vi "getAllAttributes.vi"(8 "error in (no error)":errorcluster, 11 "NativeXML in":refnum<class "NativeXML.lvclass">) -> (0 "error out":errorcluster, 1 "values":string[](array[string]), 2 "names":string[](array[string]), 3 "NativeXML out":refnum<class "NativeXML.lvclass">)   [LabVIEW 2009, in "Tools.lvlib" / "xml.lvlib" / "NativeXML.lvclass"]
uses:
  NativeXML.lvclass
  NativeXML.lvclass/NativeXML.ctl
  <vilib>/xml/Close Reference(NNMap).vi
  <vilib>/xml/Close Reference(Node).vi
  Program Files/National Instruments/LabVIEW 2009/resource/objmgr/DOMUserDefRef.rc
  <vilib>/xml/NI_XML.lvlib
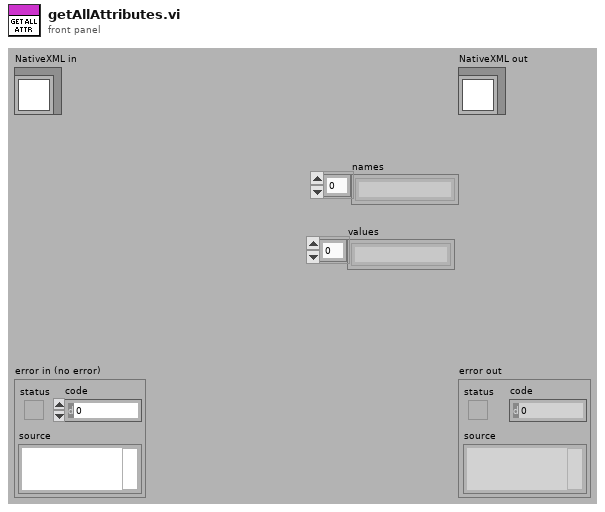
[diagram p1: front panel]
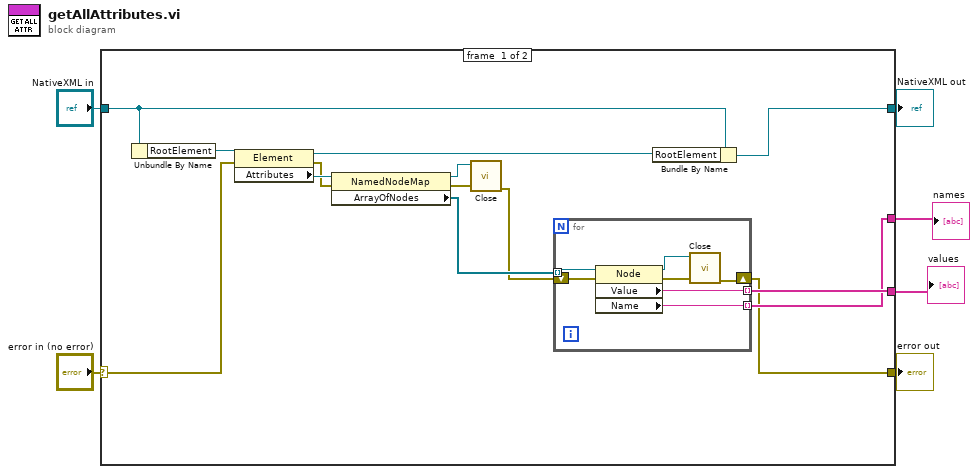
[diagram p0: block diagram]
diagram:
  n1 = case shown="No Error" "error in (no error)" {
    selector: "error in (no error)" -> [w12 w29]
    tunnel: [w14 w29] -> w5
    tunnel: [w19 w28] -> w3
    tunnel: "NativeXML in" -> [w20 w28]
    tunnel: [w18 _] -> w1
    tunnel: [w17 _] -> w2
    frame #0 {
      n2 = Unbundle By Name(w20) -> ("RootElement"=w16:refnum<k20>)
      n3 = property class="Element"(reference=w16, error in=w12) -> (reference out=w11:refnum<k20>, error out=w10:errorcluster, "Attributes"=w15:refnum<k20>)
      n4 = property class="NamedNodeMap"(reference=w15, error in=w10) -> (reference out=w8:refnum<k20>, error out=w9:errorcluster, "ArrayOfNodes"=w13:refnum<k20>[])
      n5 = call-poly <vilib>:"Close.vi"("error in (no error)"=w9, "named node map"=w8) -> ("error out"=w7:errorcluster)  [unwired: 7 in]
      n6 = for {
        tunnel: w13 -> [w27] mode=indexing
        tunnel: [w26] -> w18 mode=indexing
        tunnel: [w25] -> w17 mode=indexing
        shift-right: [w21] -> w14
        shift-left: w7 -> [w24]
        n7 = property class="Node"(reference=w27, error in=w24) -> (reference out=w22:refnum<k20>, error out=w23:errorcluster, "Value"=w26:string, "Name"=w25:string)
        n8 = call-poly <vilib>:"Close.vi"("error in (no error)"=w23, "node"=w22) -> ("error out"=w21:errorcluster)  [unwired: 7 in]
      }
      n9 = Bundle By Name(cluster=w20, "RootElement"=w11) -> (w19:refnum<class "NativeXML.lvclass">)
    }
    frame #1 {
    }
  }
  "error out" <- w5
  "NativeXML out" <- w3
  "values" <- w1
  "names" <- w2
